vi "CalcMAT_from_az_el_scale.vi"(9 "Azimuth(deg)":dbl, 10 "Elevation (deg)":dbl, 11 "Scale":dbl) -> (3 "A":T1)   [LabVIEW 2011]
doc: "This function (vi) generates a transformation matrix that contains uniform scales and Z-Y rotations. point will be scaled by Scale and rotated about Z and rotated Y axis by Azimuth and Elevation respectively. Additional rotation about X or rotated Z axis not performed by this function.\n\nThis is used to perform transformation of sessions for test perposes."
uses:
  <vilib>/Analysis/Matrix/Datatypes/RealMatrix.ctl
  <vilib>/Analysis/Matrix/Numeric/Multiply/Multiply - R,RM.vi
  <vilib>/Analysis/Matrix/NI_Matrix.lvlib
panel:
  in  "barrel_rotation(deg)":dbl
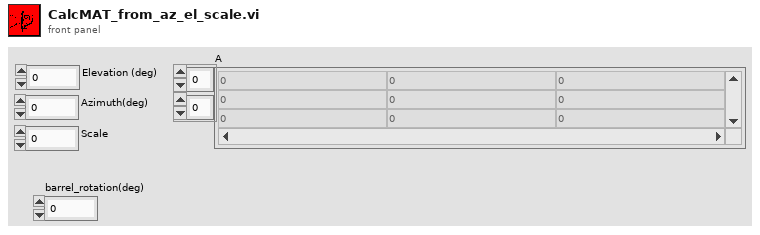
[diagram p1: front panel]
types:
  T1 = typedef "NI_Matrix.lvlib/RealMatrix.ctl" = dbl[][]
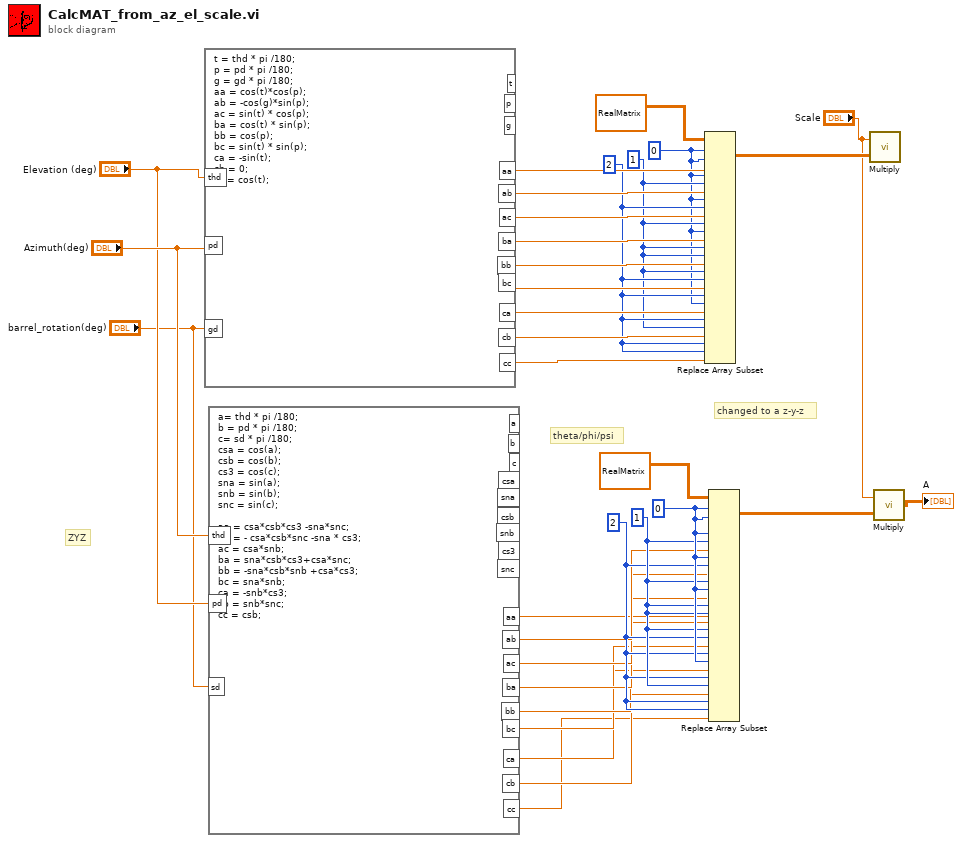
[diagram p0: block diagram]
diagram:
  w16 = 2 ("disabled index (row)")
  w17 = 1 ("disabled index (row)")
  w18 = 0 ("index (row)")
  w23 = 2 ("disabled index (row)")
  w22 = 1 ("disabled index (row)")
  w21 = 0 ("index (row)")
  # "changed to a z-y-z"
  # "ZYZ"
  # "theta/phi/psi"
  n1 = formula code="t = thd * pi /180;\np = pd * pi /180;\ng = gd * pi /180;\naa = cos(t)*cos(p);\nab = -cos(g)*sin(p);\nac = sin(t) * cos(p);\nba = cos(t) * sin(p);\nbb = cos(p);\nbc = sin(t) * sin(p);\nca = -sin(t);\ncb = 0;\ncc = cos(t);"("thd"="Elevation (deg)", "pd"="Azimuth(deg)", "gd"="barrel_rotation(deg)") -> ("aa"=w25:dbl, "ab"=w24:dbl, "ac"=w26:dbl, "ba"=w27:dbl, "bb"=w28:dbl, "bc"=w29:dbl, "ca"=w30:dbl, "cb"=w31:dbl, "cc"=w32:dbl)  [unwired: 3 out]
  n2 = formula code="a= thd * pi /180;\nb = pd * pi /180;\nc= sd * pi /180;\ncsa = cos(a);\ncsb = cos(b);\ncs3 = cos(c);\nsna = sin(a);\nsnb = sin(b);\nsnc = sin(c);\n\naa = csa*csb*cs3 -sna*snc;\nab = - csa*csb*snc -sna * cs3;\nac = csa*snb;\nba = sna*csb*cs3+csa*snc;\nbb = -sna*csb*snb +csa*cs3;\nbc = sna*snb;\nca = -snb*cs3;\ncb = snb*snc;\ncc = csb;"("thd"="Azimuth(deg)", "pd"="Elevation (deg)", "sd"="barrel_rotation(deg)") -> ("aa"=w14:dbl, "ab"=w15:dbl, "ac"=w13:dbl, "ba"=w12:dbl, "bb"=w11:dbl, "bc"=w10:dbl, "ca"=w9:dbl, "cb"=w8:dbl, "cc"=w7:dbl)  [unwired: 9 out]
  n3 = Replace Array Subset(array=T1 [[0.999624978362674, -0.00030198578782703045, -9.190317617430166e-05], [4.163336342344337e-16, 1.0000000000000002, 5.551115123125783e-16], [1.6653345369377348e-16, 1.6653345369377348e-16, 0.9999999999999999]] ("A - Transformation Matrix"), new element #1=w25, index (row) #1=w21, index (col) #1=w21, new element #2=w24, index (row) #2=w21, index (col) #2=w22, new element #3=w26, index (row) #3=w21, index (col) #3=w23, new element #4=w27, index (row) #4=w22, index (col) #4=w21, new element #5=w28, index (row) #5=w22, index (col) #5=w22, new element #6=w29, index (row) #6=w22, index (col) #6=w23, new element #7=w30, index (row) #7=w23, index (col) #7=w21, new element #8=w31, index (row) #8=w23, index (col) #8=w22, new element #9=w32, index (row) #9=w23, index (col) #9=w23) -> (w33:T1)
  n4 = Replace Array Subset(array=T1 [[0.999624978362674, -0.00030198578782703045, -9.190317617430166e-05], [4.163336342344337e-16, 1.0000000000000002, 5.551115123125783e-16], [1.6653345369377348e-16, 1.6653345369377348e-16, 0.9999999999999999]] ("A - Transformation Matrix"), new element #1=w14, index (row) #1=w18, index (col) #1=w18, new element #2=w15, index (row) #2=w18, index (col) #2=w17, new element #3=w13, index (row) #3=w18, index (col) #3=w16, new element #4=w12, index (row) #4=w17, index (col) #4=w18, new element #5=w11, index (row) #5=w17, index (col) #5=w17, new element #6=w10, index (row) #6=w17, index (col) #6=w16, new element #7=w9, index (row) #7=w16, index (col) #7=w18, new element #8=w8, index (row) #8=w16, index (col) #8=w17, new element #9=w7, index (row) #9=w16, index (col) #9=w16) -> (w6:T1)
  n5 = call-poly <vilib>:"Multiply.vi"("Real Matrix A"=w33, "Real Scalar c"="Scale") -> ()  [unwired: 1 out]
  n6 = call-poly <vilib>:"Multiply.vi"("Real Matrix A"=w6, "Real Scalar c"="Scale") -> ("c * A"=→"A":T1)
